vi "Const Sizes.vi"() -> (3 "Sizes":T1)   [LabVIEW 2020, in "FlexBlock.xnode"]
uses:
  FlexBlock.xnode
  FlexBlocks/Size Constants.ctl
  FlexBlocks/FlexBlocks.lvlib
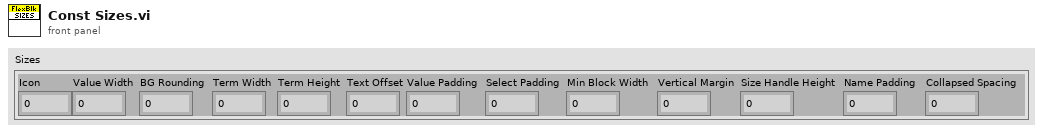
[diagram p1: front panel]
types:
  T1 = typedef "FlexBlocks.lvlib/Size Constants.ctl" = cluster{"Icon":i32, "Value Width":i32, "BG Rounding":i32, "Term Width":i32, "Term Height":i32, "Text Offset":i32, "Value Padding":i32, "Select Padding":i32, "Min Block Width":i32, "Vertical Margin":i32, "Size Handle Height":i32, "Name Padding":i32, "Collapsed Spacing":i32}
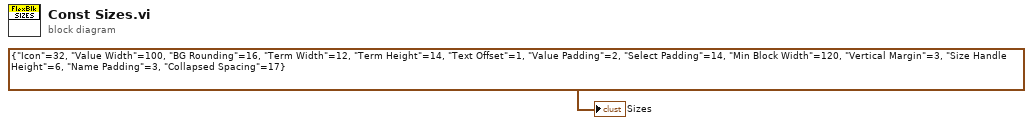
[diagram p0: block diagram]
diagram:
  "Sizes" <- T1 {"Icon"=32, "Value Width"=100, "BG Rounding"=16, "Term Width"=12, "Term Height"=14, "Text Offset"=1, "Value Padding"=2, "Select Padding"=14, "Min Block Width"=120, "Vertical Margin"=3, "Size Handle Height"=6, "Name Padding"=3, "Collapsed Spacing"=17} ("Sizes")
